vi "GUI.Button.SetText.vi"(7 "referenceToControls in":refnum<vi>[](array[refnum]), 8 "error in (no error)":errorcluster, 10 "buttonText":string, 11 "buttonName":string) -> (0 "error out":errorcluster, 5 "referenceToControls out":refnum<vi>[](array[refnum]))   [LabVIEW 2019]
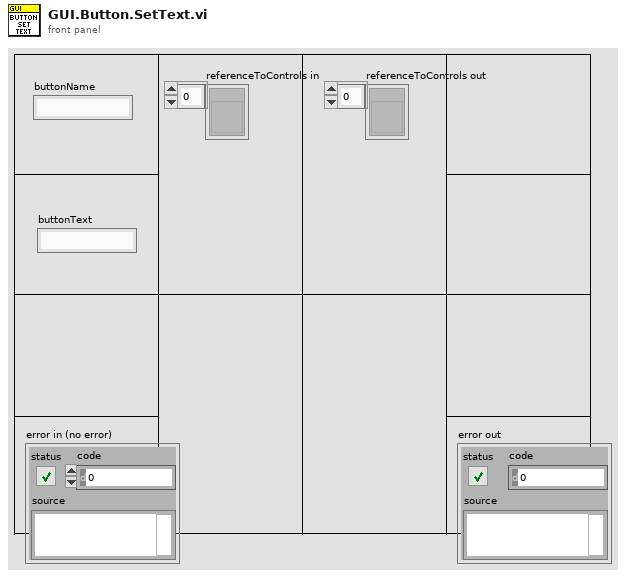
[diagram p1: front panel]
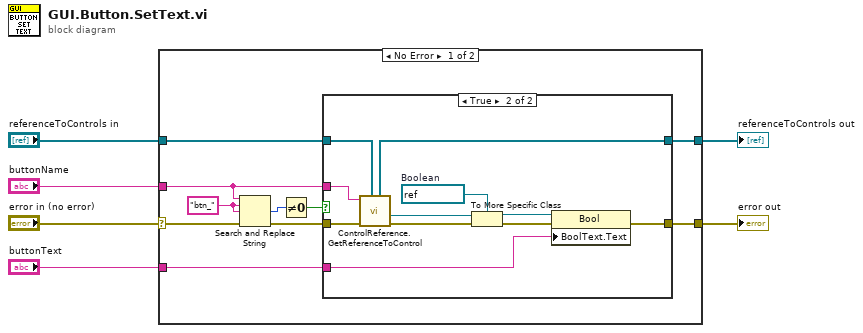
[diagram p0: block diagram]
diagram:
  n1 = case shown="No Error" "error in (no error)" {
    selector: "error in (no error)" -> [w13 w31]
    tunnel: [w16 w31] -> w4
    tunnel: "buttonName" -> [w11 _]
    tunnel: "referenceToControls in" -> [w8 w30]
    tunnel: "buttonText" -> [w15 _]
    tunnel: [w7 w30] -> w1
    frame No Error {
      w14 = "btn_"
      n2 = Search and Replace String(input string=w11, search string=w14, replace string=w14, error in=w13) -> (number of replacements=w10:i32, error out=w12:errorcluster)  [unwired: 4 in, 2 out]
      n3 = Not Equal To 0?(x=w10) -> (x != 0?=w9:bool)
      n4 = case shown="True" w9 {
        tunnel: w12 -> [w18 w23]
        tunnel: w8 -> [w17 w22]
        tunnel: w11 -> [_ w21]
        tunnel: [w18 w25] -> w16
        tunnel: w15 -> [_ w24]
        tunnel: [w17 w19] -> w7
        frame False {
        }
        frame True {
          w28 = refnum<vi> refnum  # Boolean
          n5 = call "ControlReference.GetReferenceToControl.vi"("referenceToControls in"=w22, "error in (no error)"=w23, "controlLabelText"=w21) -> ("error out"=w26:errorcluster, "referenceToControl"=w20:refnum<vi>, "referenceToControls out"=w19:refnum<vi>[])  [unwired: 6 in]
          n6 = To More Specific Class(target class=w28, reference=w20, error in=w26) -> (specific class reference=w27:refnum<vi>, error out=w29:errorcluster)
          n7 = property class="Bool"(reference=w27, error in=w29, "BoolText.Text"=w24) -> (error out=w25:errorcluster)  [unwired: 1 out]
        }
      }
    }
    frame Error {
    }
  }
  "error out" <- w4
  "referenceToControls out" <- w1
